vi "Optimiser SBlock Creator.vi"(8 "Common Parameters":T1[](array[typedef]), 9 "Number of repetitions":u16, 10 "Script Path":path, 11 "FPGA Name":string) -> (0 "error out":errorcluster, 2 "Schedule Block out":refnum<class "Schedule Block.lvclass">)   [LabVIEW 2020, in "CIRCUS_uServices.lvlib" / "Scheduler.lvlib"]
uses:
  Scheduler.lvlib
  Run Utilities/Schedule Block/Schedule Block.lvclass
  Run Utilities/Optimiser SBlock/Optimiser SBlock.lvclass
  Run Utilities/Run Instance/Run Instance.lvclass
  Run Utilities/Schedule Block/Create SBlock (array of pairs).vi
  Run Utilities/Optimiser Cell/Optimiser Cell.lvclass
  C:/Users/marco/Documents/GitHub_Lab/CIRCUS/CIRCUS uServices et al/Run Utilities/Schedule Block/Schedule Block.lvclass
  C:/Users/marco/Documents/GitHub_Lab/CIRCUS/CIRCUS uServices et al/Run Utilities/Optimiser SBlock/Optimiser SBlock.lvclass
  Run Utilities/Scan SBlock/Parameter name with value - GUI.ctl
  Run Utilities/Scan SBlock/Scan SBlock.lvclass
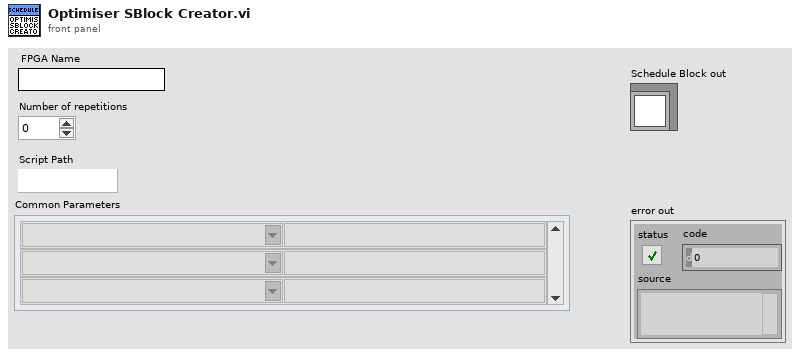
[diagram p1: front panel]
types:
  T1 = typedef "CIRCUS_uServices.lvlib/Run Utilities.lvlib/Scan SBlock.lvclass/Parameter name with value - GUI.ctl" = cluster{"Parameter Name":string, "Parameter Value":string}
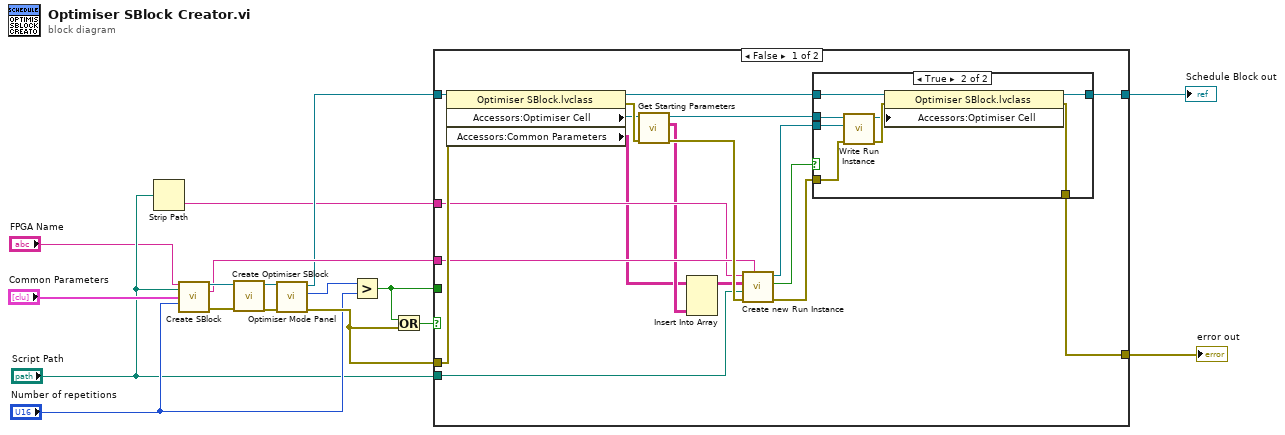
[diagram p0: block diagram]
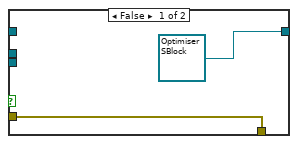
[diagram p2: hidden frame]
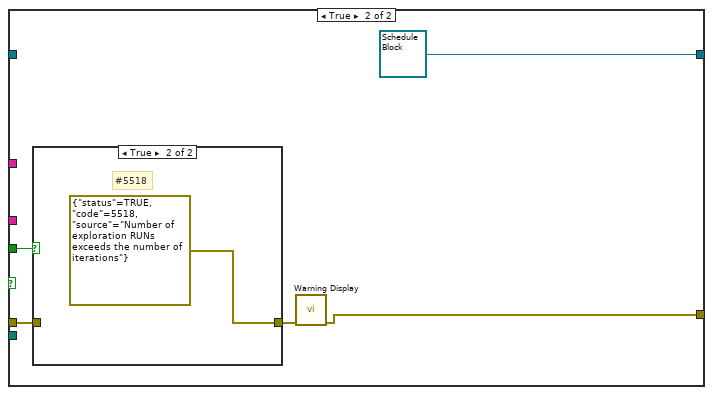
[diagram p3: hidden frame]
diagram:
  n1 = Strip Path(path="Script Path") -> (name=w2:string)  [unwired: 1 out]
  n2 = call-poly "Create SBlock.vi"("FPGA Name"="FPGA Name", "Script Path"="Script Path", "Common Parameters"="Common Parameters", "Number of repetitions"="Number of repetitions") -> ("Schedule Block out"=w17:refnum<class "Schedule Block.lvclass">, "FPGA Name"=w11:string, "error out"=w16:errorcluster)  [unwired: 9 in]
  n3 = call "Create Optimiser SBlock.vi"("error in (no error)"=w16, "Schedule Block in"=w17) -> ("error out"=w6:errorcluster, "Optimiser SBlock out"=w12:refnum<class "Optimiser SBlock.lvclass">)  [unwired: 8 in]
  n4 = call "Optimiser Mode Panel.vi"("error in (no error)"=w6, "Optimiser SBlock in"=w12) -> ("error out"=w9:errorcluster, "No. of exploration RUNs out"=w5:u32, "Optimiser SBlock out"=w7:refnum<class "Optimiser SBlock.lvclass">)  [unwired: 7 in]
  n5 = Greater?(x=w5, y="Number of repetitions") -> (0:w8:bool)
  n6 = Or(x=w8, y=w9) -> (x .or. y?=w10:bool)
  n7 = case shown="False" w10 {
    tunnel: w2 -> [w30 _]
    tunnel: "Script Path" -> [w32 _]
    tunnel: [w18 w49] -> w14
    tunnel: [w23 refnum<class "Schedule Block.lvclass"> refnum ("Schedule Block out")] -> w13
    tunnel: w11 -> [w31 _]
    tunnel: w9 -> [w34 w47]
    tunnel: w8 -> [_ w48]
    tunnel: w7 -> [w29 _]
    frame False {
      n8 = property class="Optimiser SBlock.lvclass"(reference=w29, error in=w34) -> (reference out=w24:refnum<class "Optimiser SBlock.lvclass">, error out=w33:errorcluster, "Accessors:Optimiser Cell"=w25:refnum<class "Optimiser Cell.lvclass">, "Accessors:Common Parameters"=w26:string[][])
      n9 = call-dynamic "Get Starting Parameters.vi"("error in (no error)"=w33, "Optimiser Cell in"=w25) -> ("error out"=w35:errorcluster, "Starting Values for Parameters"=w28:string[][], "Optimiser Cell out"=w22:refnum<class "Optimiser Cell.lvclass">)  [unwired: 7 in]
      n10 = Insert Into Array(array=w26, new element=w28) -> (w27:string[][])  [unwired: 2 in]
      n11 = call "Create new Run Instance.vi"("Kasli"=w31, "error in"=w35, "Script Path"=w32, "Parameters"=w27, "Script Name"=w30) -> ("error out"=w19:errorcluster, "Created?"=w21:bool, "Run Instance"=w20:refnum<class "Run Instance.lvclass">)  [unwired: 4 in]
      n12 = case shown="True" w21 {
        tunnel: w24 -> [_ w44]
        tunnel: [refnum<class "Optimiser SBlock.lvclass"> refnum ("Optimiser SBlock out") w43] -> w23
        tunnel: w22 -> [_ w42]
        tunnel: w20 -> [_ w39]
        tunnel: w19 -> [w36 w40]
        tunnel: [w36 w38] -> w18
        frame False {
        }
        frame True {
          n13 = call-dynamic "Write Run Instance.vi"("error in (no error)"=w40, "Run Instance"=w39, "Schedule Cell in"=w42) -> ("error out"=w45:errorcluster, "Schedule Cell out"=w41:refnum<class "Optimiser Cell.lvclass">)  [unwired: 7 in]
          n14 = property class="Optimiser SBlock.lvclass"(reference=w44, error in=w45, "Accessors:Optimiser Cell"=w41) -> (reference out=w43:refnum<class "Optimiser SBlock.lvclass">, error out=w38:errorcluster)
        }
      }
    }
    frame True {
      n15 = case shown="True" w48 {
        tunnel: w47 -> [w51 _]
        tunnel: [w51 errorcluster {"status"=TRUE, "code"=5518, "source"="Number of exploration RUNs exceeds the number of iterations"} ("error out")] -> w46
        frame False {
        }
        frame True {
          # "#5518"
        }
      }
      n16 = call "Warning Display.vi"("error in (no error)"=w46) -> ("error out"=w49:errorcluster)  [unwired: 10 in]
    }
  }
  "error out" <- w14
  "Schedule Block out" <- w13
